vi "Test Pics.vi"() -> ()   [LabVIEW 2020]
uses:
  <vilib>/picture/picture.llb/imagedata.ctl
  <vilib>/Utility/sysdir.llb/System Directory Type.ctl
panel:
  out "appended path 2":path
  in  "appended path 3":path
  out "appended path":path
  out "WiringRules[]":T1(array[ring])
  out "new picture 4":picture
  out "new picture 3":picture
  out "new picture 2":picture
  out "new picture":picture
  out "Get ConnPane Image":T2
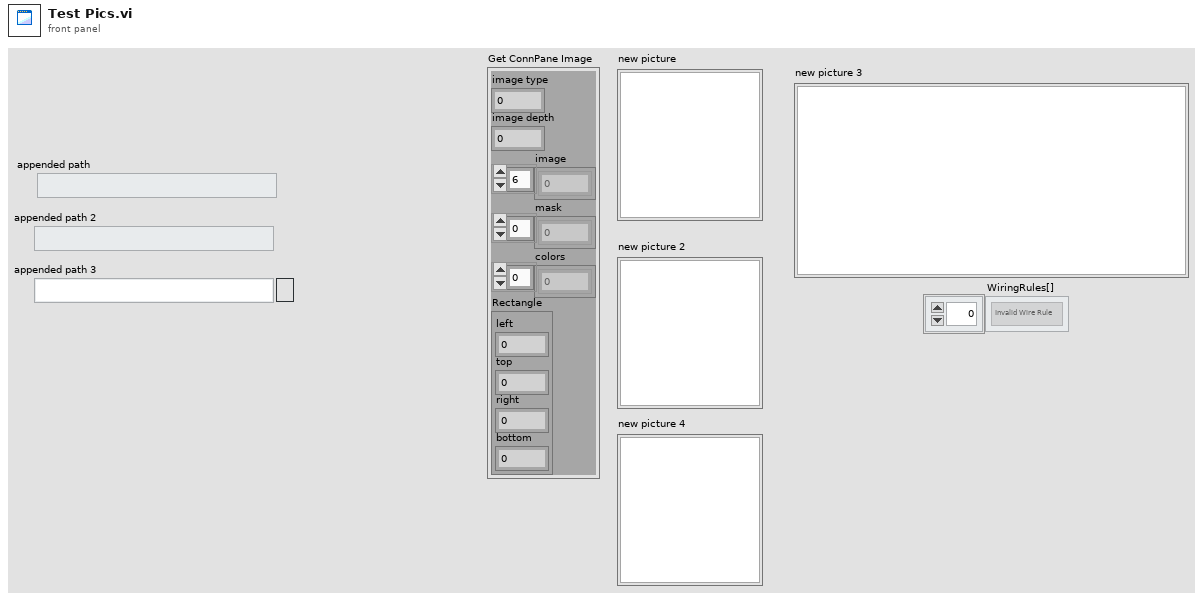
[diagram p1: front panel]
types:
  T1 = enum16{"Invalid Wire Rule", "Required", "Recommended", "Optional", "Dynamic Dispatch"}[]
  T2 = typedef "imagedata.ctl" = cluster{"image type":i32, "image depth":i32, "image":u8[], "mask":u8[], "colors":u32[], "Rectangle":cluster{"left":i16, "top":i16, "right":i16, "bottom":i16}}
  T3 = typedef "System Directory Type.ctl" = i32
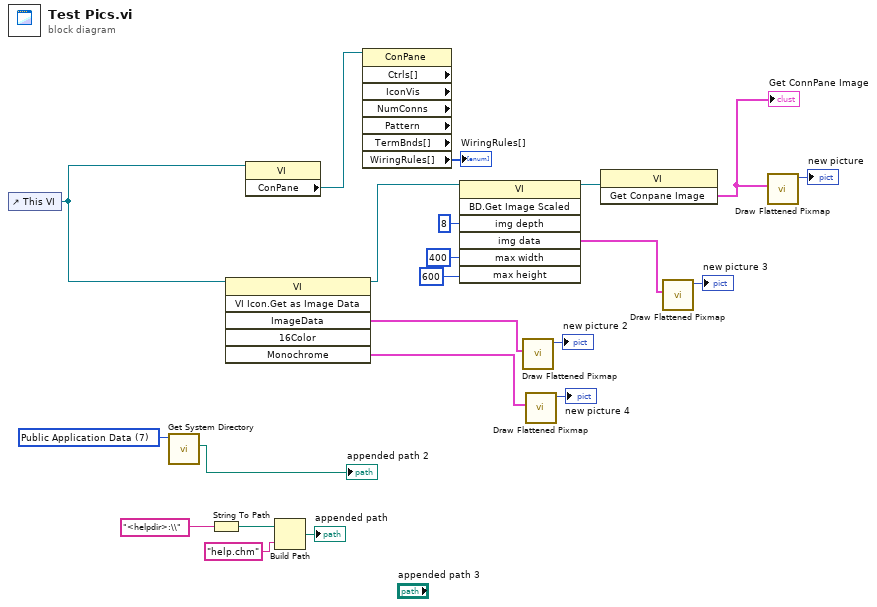
[diagram p0: block diagram]
diagram:
  w6 = T3 7 items=["User Home"=0, "User Desktop"=1, "User Documents"=2, "User Application Data"=3, "User Preferences"=4, "User Temporary"=5, "Public Documents"=6, "Public Application Data"=7, "Public Preferences"=8, "Public Cache"=13, "System Core Libraries"=9, "System Installed Libraries"=10, "Application Files"=11, "Boot Volume Root"=12] ("system directory type")
  n1 = control-ref of="This VI"() -> (w20:refnum<vi>)
  n2 = call <vilib>:"Get System Directory.vi"("system directory type"=w6) -> ("system directory"=→"appended path 2":path)  [unwired: 10 in]
  n3 = String To Path(string="<helpdir>:\\") -> (path=w2:path)
  n4 = invoke class="VI" method="VI Icon.Get as Image Data"(reference=w20) -> (reference out=w22:refnum<vi>, "ImageData"=w15:T2, "Monochrome"=w8:T2)  [unwired: 5 in, 3 out]
  n5 = property class="VI"(reference=w20) -> ("ConPane"=w19:refnum<vi>)  [unwired: 1 in, 2 out]
  n6 = Build Path(base path=w2, name or relative path="help.chm") -> (appended path=→"appended path":path)
  n7 = property class="ConPane" props=["Ctrls[]", "IconVis", "NumConns", "Pattern", "TermBnds[]", "WiringRules[]"](reference=w19) -> ("WiringRules[]"=→"WiringRules[]":T1)  [unwired: 1 in, 7 out]
  n8 = invoke class="VI" method="BD.Get Image Scaled"(reference=w22, "img depth"=8 ("Image Depth"), "max width"=400 ("Maximum Width"), "max height"=600 ("Maximum Height")) -> (reference out=w21:refnum<vi>, "img data"=w10:T2)  [unwired: 3 in, 5 out]
  n9 = call <vilib>:"Draw Flattened Pixmap.vi"("image data"=w15) -> ("new picture"=→"new picture 2":picture)  [unwired: 8 in]
  n10 = call <vilib>:"Draw Flattened Pixmap.vi"("image data"=w8) -> ("new picture"=→"new picture 4":picture)  [unwired: 8 in]
  n11 = invoke class="VI" method="Get Conpane Image"(reference=w21) -> ("Get Conpane Image"=w18:T2)  [unwired: 2 in, 2 out]
  "Get ConnPane Image" <- w18
  n12 = call <vilib>:"Draw Flattened Pixmap.vi"("image data"=w10) -> ("new picture"=→"new picture 3":picture)  [unwired: 8 in]
  n13 = call <vilib>:"Draw Flattened Pixmap.vi"("image data"=w18) -> ("new picture"=→"new picture":picture)  [unwired: 8 in]
